vi "USB2XXX_UART_WriteReadTest.vi"() -> ()   [LabVIEW 2010]
panel:
  in  "pConfig":T1={"BaudRate"=19200, "WordLength"=0, "StopBits"=0, "Parity"=0, "TEPolarity"=0}
  out "Readed Data Num":i32
  out "Read Data(Hex)":string
  in  "Write Data(Hex)":string="11 22 33 44 55 66 77 88"
  in  "Channel Index":u8(ring) items=["UART0", "UART1"]
  in  "Device Index":i32(ring) items=["0", "1", "2", "3", "4", "5"]
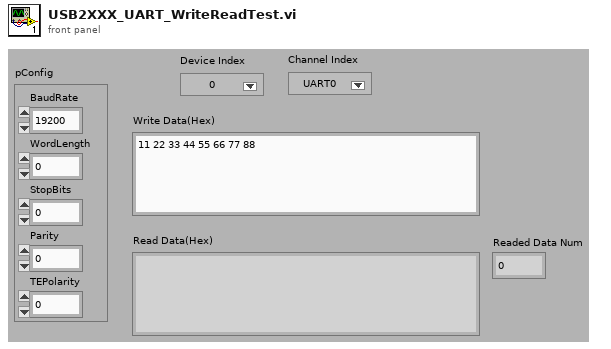
[diagram p1: front panel]
types:
  T1 = cluster{"BaudRate":u32, "WordLength":u8, "StopBits":u8, "Parity":u8, "TEPolarity":u8}
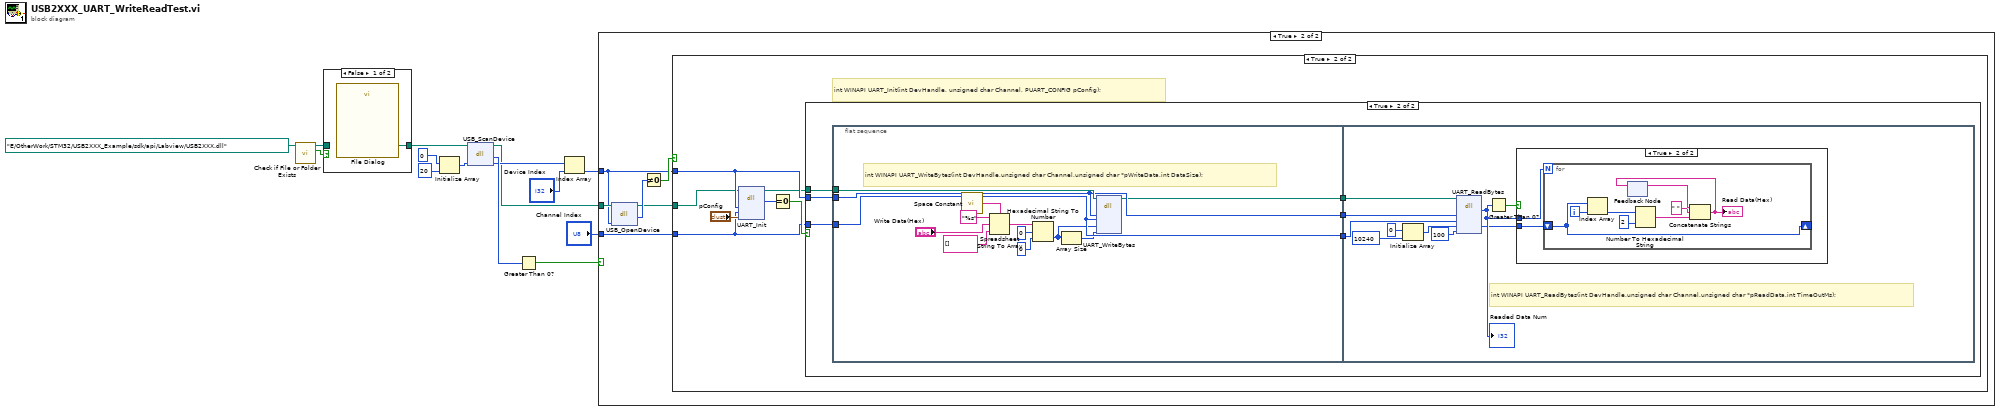
[diagram p0: block diagram]
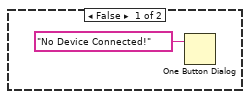
[diagram p3: hidden frame]
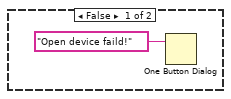
[diagram p4: hidden frame]
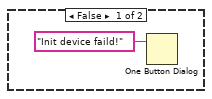
[diagram p5: hidden frame]
diagram:
  n1 = call <vilib>:"Check if File or Folder Exists.vi"("path"=path "E:/OtherWork/STM32/USB2XXX_Example/sdk/api/Labview/USB2XXX.dll" ("path in")) -> ("file or folder exists?"=w3:bool, "dup path"=w2:path)  [unwired: 8 in, 1 out]
  n2 = case shown="False" w3 {
    tunnel: w2 -> [_ w16]
    tunnel: [w15 w16] -> w1
    frame False {
      n3 = call "File Dialog"() -> ("selected path"=w15:path)  [unwired: 12 in, 3 out]
    }
    frame True {
    }
  }
  n4 = Initialize Array(0, 20 ("dimension size")) -> (w12:i32[])
  n5 = dll-call lib="E:/OtherWork/STM32/USB2XXX_Example/examples/Labview/PublicFiles/USB2XXX.dll" fn="USB_ScanDevice"(path in=w1, "pDevNum"=w12) -> (path out=w7:path, "return type"=w11:i32, "pDevNum"=w10:i32[])  [unwired: 2 in, 1 out]
  n6 = Greater Than 0?(x=w11) -> (x > 0?=w8:bool)
  n7 = Index Array(array=w10, index="Device Index") -> (element=w6:i32)
  n8 = case shown="True" w8 {
    tunnel: w7 -> [_ w23]
    tunnel: w6 -> [_ w19]
    tunnel: "Channel Index" -> [_ w18]
    frame False {
      n9 = One Button Dialog(message="No Device Connected!") -> ()  [unwired: 1 in, 1 out]
    }
    frame True {
      n10 = dll-call lib="E:/OtherWork/STM32/USB2XXX_Example/examples/Labview/PublicFiles/USB2XXX.dll" fn="USB_OpenDevice"(path in=w23, "DevIndex"=w19) -> (path out=w20:path, "return type"=w22:u8)  [unwired: 3 in, 1 out]
      n11 = Not Equal To 0?(x=w22) -> (x != 0?=w21:bool)
      n12 = case shown="True" w21 {
        tunnel: w20 -> [_ w27]
        tunnel: w19 -> [_ w29]
        tunnel: w18 -> [_ w28]
        frame False {
          n13 = One Button Dialog(message="Open device faild!") -> ()  [unwired: 1 in, 1 out]
        }
        frame True {
          # "int WINAPI UART_Init(int DevHandle, unsigned char Channel, PUART_CONFIG pConfig);"
          n14 = dll-call lib="E:/OtherWork/STM32/USB2XXX_Example/sdk/api/Labview/USB2XXX.*" fn="UART_Init"(path in=w27, "DevHandle"=w29, "Channel"=w28, "pConfig"="pConfig") -> (path out=w26:path, "return type"=w25:i32)  [unwired: 5 in, 1 out]
          n15 = Equal To 0?(x=w25) -> (x = 0?=w31:bool)
          n16 = case shown="True" w31 {
            tunnel: w26 -> [_ w38]
            tunnel: w29 -> [_ w37]
            tunnel: w28 -> [_ w36]
            frame False {
              n17 = One Button Dialog(message="Init device faild!") -> ()  [unwired: 1 in, 1 out]
            }
            frame True {
              n18 = flat-sequence {
                tunnel: w38 -> [w44]
                tunnel: w37 -> [w43]
                tunnel: w36 -> [w42]
                tunnel: [w39] -> w35
                tunnel: [w43] -> w34
                tunnel: [w42] -> w33
                tunnel: w35 -> [w58]
                tunnel: w34 -> [w57]
                tunnel: w33 -> [w56]
                frame #0 {
                  # "int WINAPI UART_WriteBytes(int DevHandle,unsigned char Channel,unsigned char *pWriteData,int DataSize);"
                  n19 = call <vilib>:"Space Constant.vi"() -> ("String"=w47:string)
                  n20 = Spreadsheet String To Array(delimiter (Tab)=w47, format string="%s", spreadsheet string="Write Data(Hex)", array type (2D Dbl)=string[] []) -> (array=w50:string[])
                  n21 = Hexadecimal String To Number(string=w50, offset=0, default (0uL)=u8 0 ("default (0 U32)")) -> (number=w41:u8[])  [unwired: 1 out]
                  n22 = Array Size(array=w41) -> (size(s)=w40:i32)
                  n23 = dll-call lib="E:/OtherWork/STM32/USB2XXX_Example/sdk/api/Labview/USB2XXX.*" fn="UART_WriteBytes"(path in=w44, "DevHandle"=w43, "Channel"=w42, "pWriteData"=w41, "DataSize"=w40) -> (path out=w39:path)  [unwired: 7 in, 1 out]
                }
                frame #1 {
                  # "int WINAPI UART_ReadBytes(int DevHandle,unsigned char Channel,unsigned char *pReadData,int TimeOutMs);"
                  n24 = Initialize Array(u8 0 ("element"), 10240 ("dimension size")) -> (w55:u8[])
                  n25 = dll-call lib="E:/OtherWork/STM32/USB2XXX_Example/sdk/api/Labview/USB2XXX.*" fn="UART_ReadBytes"(path in=w58, "DevHandle"=w57, "Channel"=w56, "pReadData"=w55, "TimeOutMs"=100) -> ("return type"=w53:i32, "pReadData"=w52:u8[])  [unwired: 5 in, 2 out]
                  "Readed Data Num" <- w53
                  n26 = Greater Than 0?(x=w53) -> (x > 0?=w61:bool)
                  n27 = case shown="True" w61 {
                    tunnel: w53 -> [_ w63]
                    tunnel: w52 -> [_ w62]
                    frame False {
                    }
                    frame True {
                      n28 = for {
                        N: w63 -> [_]
                        shift-right: [w64] -> _
                        shift-left: w62 -> [w64]
                        i -> [w71]
                        n29 = Index Array(array=w64, index=w71) -> (element=w70:u8)
                        n30 = feedback #1() -> (w68:string)  [unwired: 1 in]
                        n31 = Number To Hexadecimal String(1:i16 2 ("width (-)"), 2:w70) -> (0:w66:string)
                        n32 = Concatenate Strings(w68, " " ("string"), w66) -> (w65:string)
                        "Read Data(Hex)" <- w65
                        n33 = feedback-in #1(w65) -> ()
                      }
                    }
                  }
                }
              }
            }
          }
        }
      }
    }
  }
